vi "显示螺丝所附点位序号.vi"(7 "Font, Size & Style":T1={"Desired Font (Application)"=enum."User-specified Font", "[User-specified Font]"={"Font Name"="", "Size"=40, "Strikeout?"=FALSE, "Italic?"=FALSE, "Underline?"=FALSE, "Outline?"=FALSE, "Shadow?"=FALSE, "Bold?"=FALSE, "Rotation Angle"=0.0}, "Horizontal Alignment"=0, "Vertical Alignment"=0} {"Horizontal Alignment" items=["Left", "Center", "Right"]; "Vertical Alignment" items=["Bottom", "Top", "Baseline"]}, 8 "显示坐标":cluster{dbl, "Numeric":dbl}[](array[cluster]), 9 "颜色":u32[](array[colorbox]), 10 "待写入数据":dbl[](array[numeric]), 11 "Img输入":T2) -> (3 "Img输出":T2)   [LabVIEW 2014]
uses:
  Global.vi
  <vilib>/vision/Image Controls.llb/IMAQ Image.ctl
panel:
  in  "Font, Size & Style 2":T1={"Desired Font (Application)"=enum."User-specified Font", "[User-specified Font]"={"Font Name"="", "Size"=30, "Strikeout?"=FALSE, "Italic?"=FALSE, "Underline?"=FALSE, "Outline?"=FALSE, "Shadow?"=FALSE, "Bold?"=FALSE, "Rotation Angle"=0.0}, "Horizontal Alignment"=0, "Vertical Alignment"=0} {"Horizontal Alignment" items=["Left", "Center", "Right"]; "Vertical Alignment" items=["Bottom", "Top", "Baseline"]}
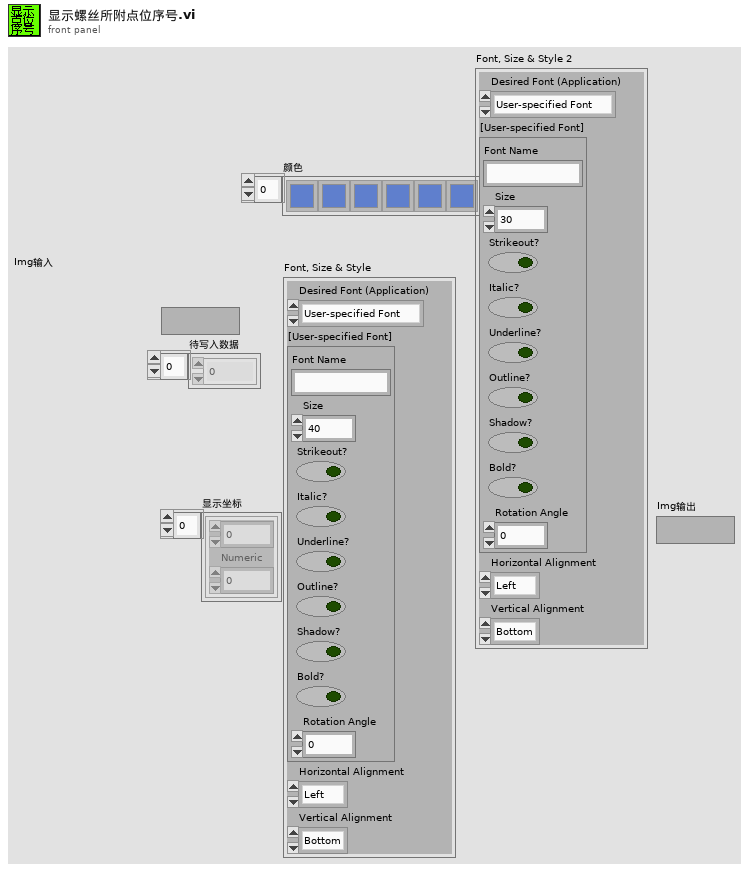
[diagram p1: front panel]
types:
  T1 = cluster{"Desired Font (Application)":enum16{"User-specified Font", "Application Font", "System Font", "Dialog Font"}, "[User-specified Font]":cluster{"Font Name":string, "Size":i16, "Strikeout?":bool, "Italic?":bool, "Underline?":bool, "Outline?":bool, "Shadow?":bool, "Bold?":bool, "Rotation Angle":dbl}, "Horizontal Alignment":i16, "Vertical Alignment":i16}
  T2 = typedef "IMAQ Image.ctl" = refnum<image>
  T3 = typedef "ModeEditeControl.ctl" = cluster{"AllModelFold":path, "AllModelNamePath":path, "所有零件型号":string[], "当前零件型号":string, "所有建立零件信息":string[][], "当前零件序号":i32, "当前产品信息":T4}
  T4 = typedef "ModelInfo.ctl" = cluster{"产品型号":string, "二维码拍照":u32, "Mark点拍照":u32}
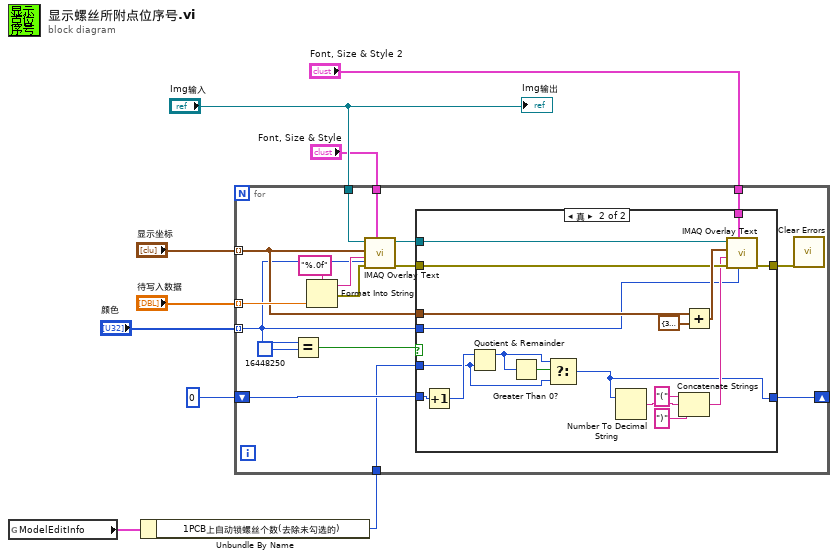
[diagram p0: block diagram]
diagram:
  n1 = global read "Global.vi" "ModelEditInfo"() -> (w2:T3)
  n2 = Unbundle By Name(w2) -> ("1PCB上自动锁螺丝个数(去除未勾选的)"=w1:i32)
  n3 = for {
    tunnel: "Img输入" -> [w26]
    tunnel: "待写入数据" -> [w25] mode=indexing
    tunnel: "显示坐标" -> [w18] mode=indexing
    tunnel: "Font, Size & Style" -> [w24]
    tunnel: "颜色" -> [w15] mode=indexing
    tunnel: "Font, Size & Style 2" -> [w20]
    shift-right: [w11] -> _
    shift-left: 0 -> [w13]
    tunnel: w1 -> [w10]
    n4 = Equal?(x=w15, y=u32 16448250 ("Text Color (black)")) -> (x = y?=w12:bool)
    n5 = Format Into String(format string="%.0f" ("格式字符串"), w25) -> (resulting string=w23:string, error out=w21:errorcluster)  [unwired: 2 in]
    n6 = call "IMAQ Overlay Text"("Text Color (black)"=w15, "Font, Size & Style"=w24, "error in (no error)"=w21, "String"=w23, "Origin"=w18, "Image"=w26) -> ("error out"=w17:errorcluster, "Image Out"=w19:T2)  [unwired: 4 in]
    n7 = case shown="真" w12 {
      tunnel: w20 -> [_ w46]
      tunnel: w19 -> [_ w45]
      tunnel: w18 -> [_ w44]
      tunnel: w17 -> [w27 w41]
      tunnel: [w27 w40] -> w16
      tunnel: w15 -> [_ w35]
      tunnel: w13 -> [w28 w32]
      tunnel: [w28 w29] -> w11
      tunnel: w10 -> [_ w30]
      frame False {
      }
      frame True {
        n8 = Increment(x=w32) -> (x+1=w31:i32)
        n9 = Quotient & Remainder(x=w31, y=w30) -> (x-y*floor(x/y)=w34:i32)  [unwired: 1 out]
        n10 = Greater Than 0?(x=w34) -> (x > 0?=w33:bool)
        n11 = Select(t=w34, s=w33, f=w30) -> (s? t:f=w29:i32)
        n12 = Number To Decimal String(number=w29) -> (decimal integer string=w39:string)  [unwired: 1 in]
        n13 = Concatenate Strings("(" ("字符串"), w39, ")" ("字符串")) -> (w36:string)
        n14 = Add(x=w44, y=cluster{dbl, "Numeric":dbl} {36.0, "Numeric"=0.0}) -> (x+y=w42:cluster{dbl, "Numeric":dbl})
        n15 = call "IMAQ Overlay Text"("Text Color (black)"=w35, "Font, Size & Style"=w46, "error in (no error)"=w41, "String"=w36, "Origin"=w42, "Image"=w45) -> ("error out"=w40:errorcluster)  [unwired: 4 in, 1 out]
      }
    }
    n16 = call <vilib>:"Clear Errors.vi"("error in (no error)"=w16) -> ()  [unwired: 5 in, 2 out]
  }
  "Img输出" <- "Img输入"
